vi "VoutVin Sub VI (FINAL).vi"(1 "error in (no error)":errorcluster, 2 "VISA Refnum in":refnum<visa-resource-name>) -> (0 "error out":errorcluster, 3 "Numeric":dbl)   [LabVIEW 2017]
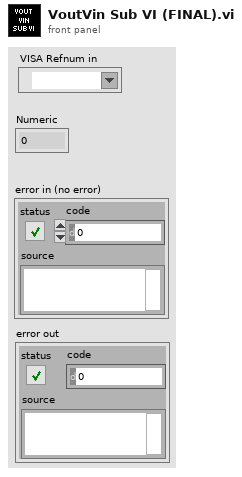
[diagram p1: front panel]
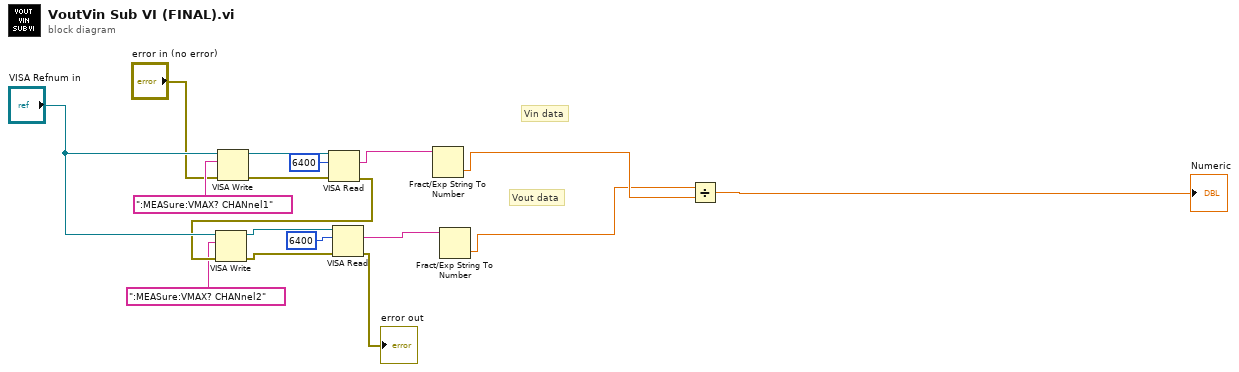
[diagram p0: block diagram]
diagram:
  # "Vin data"
  # "Vout data"
  n1 = VISA Write(VISA resource name="VISA Refnum in", write buffer=":MEASure:VMAX? CHANnel1", error in (no error)="error in (no error)") -> (VISA resource name out=w4:refnum<visa-resource-name>, error out=w6:errorcluster)  [unwired: 1 out]
  n2 = VISA Read(VISA resource name=w4, byte count=u32 6400, error in (no error)=w6) -> (read buffer=w9:string, error out=w7:errorcluster)  [unwired: 2 out]
  n3 = VISA Write(VISA resource name="VISA Refnum in", write buffer=":MEASure:VMAX? CHANnel2", error in (no error)=w7) -> (VISA resource name out=w5:refnum<visa-resource-name>, error out=w8:errorcluster)  [unwired: 1 out]
  n4 = VISA Read(VISA resource name=w5, byte count=u32 6400, error in (no error)=w8) -> (read buffer=w10:string, error out=→"error out":errorcluster)  [unwired: 2 out]
  n5 = Fract/Exp String To Number(string=w9) -> (number=w14:dbl)  [unwired: 3 in, 1 out]
  n6 = Fract/Exp String To Number(string=w10) -> (number=w13:dbl)  [unwired: 3 in, 1 out]
  n7 = Divide(x=w13, y=w14) -> (x/y=→"Numeric":dbl)
